vi "dvr_get.vi"(8 "error in (no error)":errorcluster, 11 "OSA300 in":refnum<class "OSA300.lvclass">) -> (0 "error out":errorcluster, 2 "data value ref":T1, 3 "OSA300 out":refnum<class "OSA300.lvclass">)   [LabVIEW 2010, in "OSA300.lvclass"]
uses:
  OSA300.lvclass
  OSA300_DVR.ctl
  OSA300_data.ctl
  _OSAchannel_class/OSAchannel.lvclass
  _misc/Thorlabs_FTS_misc.llb/channelType_spectrum.ctl
  OSA300.lvclass/OSA300.ctl
  OSA20X_misc.lvlib
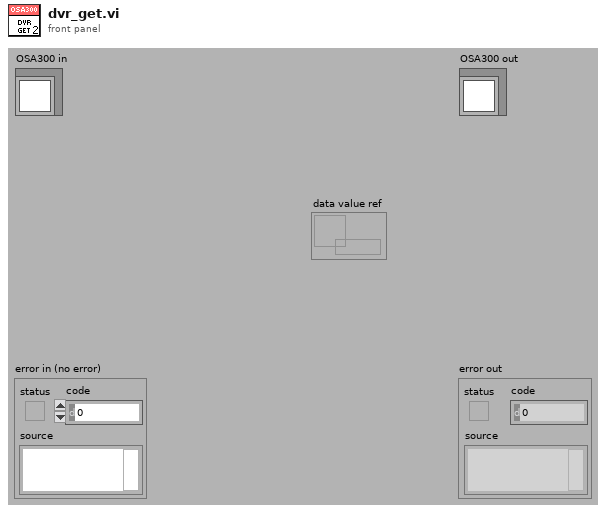
[diagram p1: front panel]
types:
  T1 = typedef "OSA300.lvclass/OSA300_DVR.ctl" = refnum<data-value>
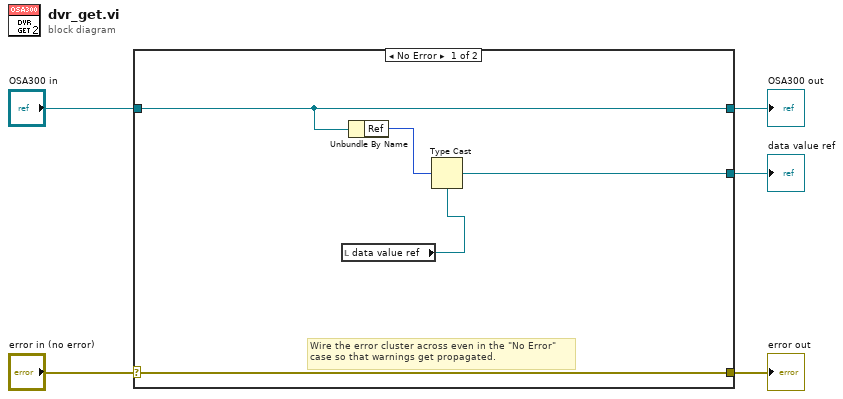
[diagram p0: block diagram]
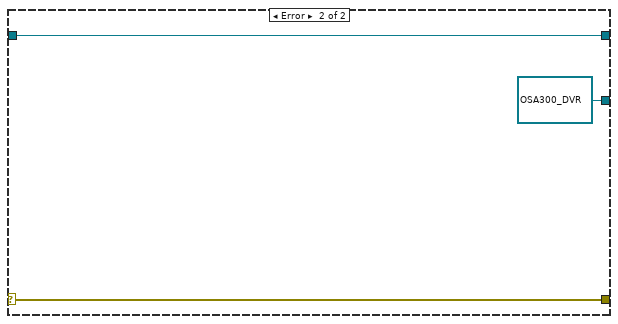
[diagram p2: hidden frame]
diagram:
  n1 = case shown="No Error" "error in (no error)" {
    selector: "error in (no error)" -> [w10 w13]
    tunnel: [w10 w13] -> w4
    tunnel: [w8 w12] -> w2
    tunnel: "OSA300 in" -> [w8 w12]
    tunnel: [w7 T1 refnum ("data value reference 2")] -> w1
    frame No Error {
      # "Wire the error cluster across even in the \"No Error\"\ncase so that warnings get propagated."
      n2 = local read "data value ref"() -> (w6:T1)
      n3 = Unbundle By Name(w8) -> ("Ref"=w9:u32)
      n4 = Type Cast(type=w6, x=w9) -> (*(type *) &x=w7:T1)
    }
    frame Error {
    }
  }
  "error out" <- w4
  "OSA300 out" <- w2
  "data value ref" <- w1
